vi "Controller - Fire Update Data.vi"(8 "error in (no error)":errorcluster, 9 "Numeric":dbl, 10 "Blink CNTRLR2":bool, 11 "View Model":T1) -> (0 "error out":errorcluster)   [LabVIEW 2017]
doc: "Generate user event from controller for update HostView data."
uses:
  View Model/Controls/View Model.ctl
  View Model/Controls/Shared Model.ctl
  Error Handler/Controls/Error Model.ctl
  Error Handler/Controls/Error Event.ctl
  Error Handler/Controls/Error Type.ctl
  Controls/Controller Model.ctl
  Controls/Controller Event.ctl
  Controls/Controller Command.ctl
  Controls/Controller Overhead.ctl
  Real-Time/RT Status.ctl
  Real-Time/RT Loop Status.ctl
  Controls/Controller Update Data.ctl
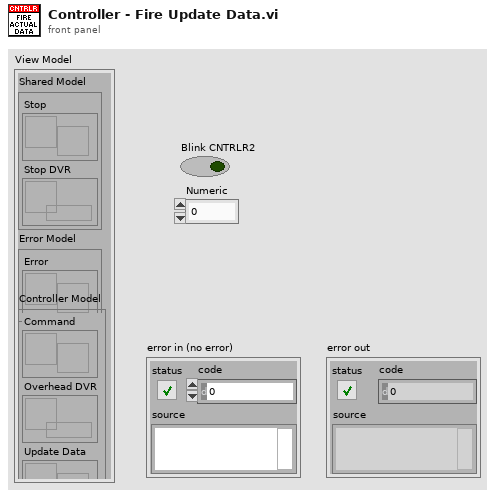
[diagram p1: front panel]
types:
  T1 = typedef "View Model.ctl" = cluster{"Shared Model":T2, "Error Model":T3, "Controller Model":T4}
  T2 = typedef "Shared Model.ctl" = cluster{"Stop":refnum<user-event>, "Stop DVR":refnum<data-value>}
  T3 = typedef "Error Model.ctl" = cluster{"Error":refnum<user-event>}
  T4 = typedef "Controller Model.ctl" = cluster{"Command":refnum<user-event>, "Overhead DVR":refnum<data-value>, "Update Data":refnum<user-event>}
  T5 = typedef "Controller Update Data.ctl" = cluster{"Blink CNTRLR2":bool, "Numeric":dbl}
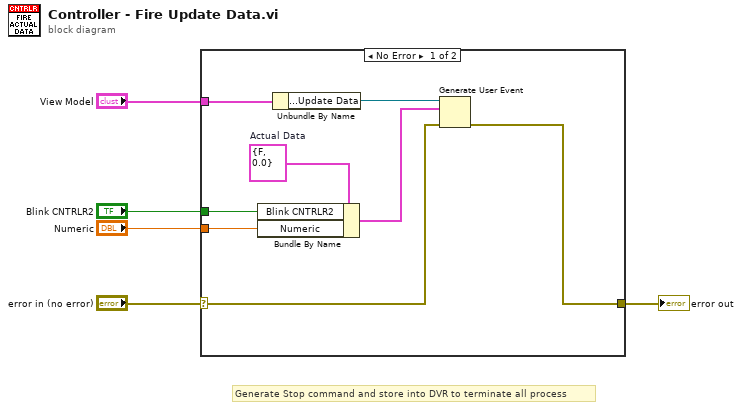
[diagram p0: block diagram]
diagram:
  # "Generate Stop command and store into DVR to terminate all process"
  n1 = case shown="No Error" "error in (no error)" {
    selector: "error in (no error)" -> [w12 w14]
    tunnel: [w11 w14] -> w4
    tunnel: "View Model" -> [w10 _]
    tunnel: "Numeric" -> [w7 _]
    tunnel: "Blink CNTRLR2" -> [w6 _]
    frame No Error {
      w9 = T5 {"Blink CNTRLR2"=FALSE, "Numeric"=0.0}  # Actual Data
      n2 = Bundle By Name(cluster=w9, "Blink CNTRLR2"=w6, "Numeric"=w7) -> (w8:T5)
      n3 = Unbundle By Name(w10) -> ("Controller Model.Update Data"=w13:refnum<user-event>)
      n4 = Generate User Event(user event=w13, event data cluster=w8, error in=w12) -> (error out=w11:errorcluster)  [unwired: 1 in, 1 out]
    }
    frame Error {
    }
  }
  "error out" <- w4
